vi "Add Wfm Header.vi"(8 "error in (no error)":errorcluster, 9 "Wfm Header":T1, 10 "Metadata":string, 11 "TCP Writer in":refnum<class "TCP Writer.lvclass">) -> (0 "error out":errorcluster, 3 "TCP Writer out":refnum<class "TCP Writer.lvclass">)   [LabVIEW 2012, in "TCP Classes.lvlib" / "TCP Writer.lvclass"]
uses:
  TCP Writer.lvclass
  Common/Controls/Waveform Header.ctl
  TCP Writer.lvclass/TCP Writer.ctl
  Common/Controls/Waveform Header with Enbl.ctl
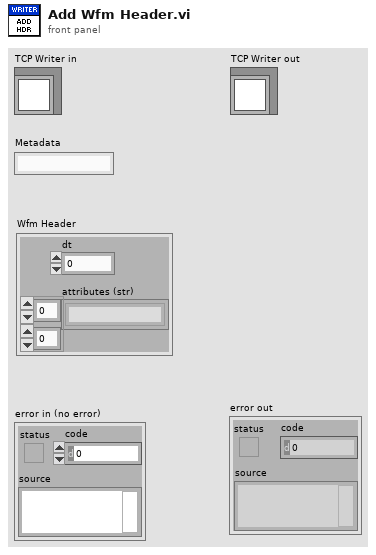
[diagram p1: front panel]
types:
  T1 = typedef "Waveform Header.ctl" = cluster{"dt":dbl, "attributes (str)":string[][]}
  T2 = typedef "Waveform Header with Enbl.ctl" = cluster{"Send Wfm Hdr?":bool, "Wfm Header":T1}
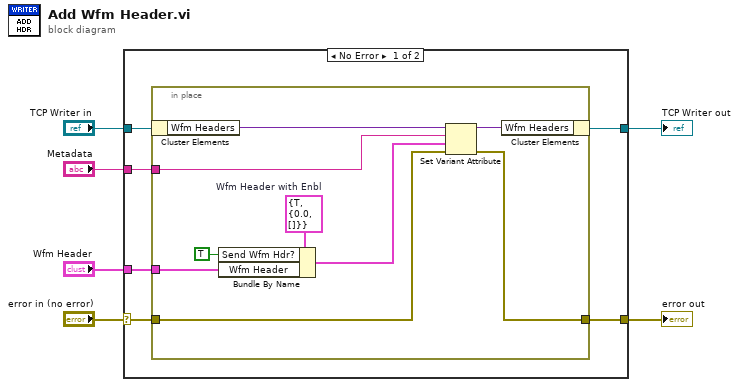
[diagram p0: block diagram]
diagram:
  n1 = case shown="No Error" "error in (no error)" {
    selector: "error in (no error)" -> [w8 w23]
    tunnel: [w7 w23] -> w5
    tunnel: [w10 w22] -> w3
    tunnel: "TCP Writer in" -> [w12 w22]
    tunnel: "Wfm Header" -> [w11 _]
    tunnel: "Metadata" -> [w9 _]
    frame No Error {
      n2 = in-place {
        in-place-border: w11 -> [w20]
        in-place-border: w9 -> [w15]
        in-place-border: w8 -> [w14]
        in-place-border: [w13] -> w7
        w21 = T2 {"Send Wfm Hdr?"=TRUE, "Wfm Header"={"dt"=0.0, "attributes (str)"=[]}}  # Wfm Header with Enbl
        n3 = in-place-cluster #1(w12) -> ("Wfm Headers"=w18:variant)
        n4 = Bundle By Name(cluster=w21, "Send Wfm Hdr?"=TRUE, "Wfm Header"=w20) -> (w16:T2)
        n5 = Set Variant Attribute(Variant=w18, name=w15, value=w16, error in=w14) -> (Variant out=w17:variant, error out=w13:errorcluster)  [unwired: 1 out]
        n6 = in-place-cluster #1("Wfm Headers"=w17) -> (w10:refnum<class "TCP Writer.lvclass">)
      }
    }
    frame Error {
    }
  }
  "error out" <- w5
  "TCP Writer out" <- w3
